vi "uploadProg.vi"(11 "editArray":T1[](array[typedef])) -> (0 "error out":errorcluster)   [LabVIEW 2014]
uses:
  typeDefs/editControl.ctl
  typeDefs/variantFlat.ctl
  typeDefs/pixxelAction.ctl
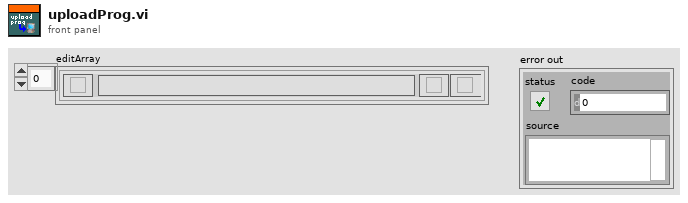
[diagram p1: front panel]
types:
  T1 = typedef "editControl.ctl" = cluster{"edit":bool, "info":string, "variantFlat":T2, "codeCluster":cluster{"code":u8[][]}, "del":bool, "ins":bool}
  T2 = typedef "variantFlat.ctl" = cluster{"type string":i16[], "data string":string}
  T3 = typedef "pixxelAction.ctl" = enum16{"init", "watchdog", "headScene", "setPixel", "tailScene", "headProg", "tailProg", "showSceneFrame", "black", "playFrames", "close", "uploadProg", "startProg", "pauseProg", "stopProg", "jumpTo", "setIP", "setGW", "initFlash", "saveScene", "saveProgram"}
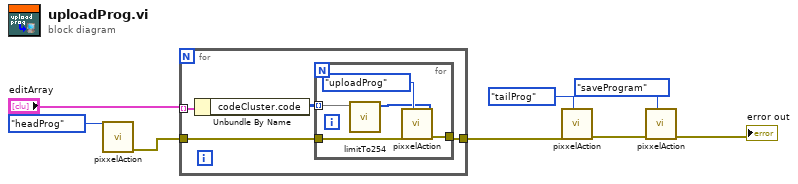
[diagram p0: block diagram]
diagram:
  n1 = call "pixxelAction.vi"("PIXXELaction"=pixxelAction."headProg") -> ("error out"=w5:errorcluster)  [unwired: 10 in]
  n2 = for {
    tunnel: [w12] -> w7
    tunnel: "editArray" -> [w11] mode=indexing
    tunnel: w5 -> [w9]
    n3 = Unbundle By Name(w11) -> ("codeCluster.code"=w10:u8[][])
    n4 = for {
      tunnel: [w17] -> w12
      tunnel: w10 -> [w15] mode=indexing
      tunnel: w9 -> [w13]
      n5 = call "limitTo254.vi"("params"=w15) -> ("limitedTo254"=w14:u8[])  [unwired: 10 in]
      n6 = call "pixxelAction.vi"("inputArray"=w14, "PIXXELaction"=pixxelAction."uploadProg", "error in (no error)"=w13) -> ("error out"=w17:errorcluster)  [unwired: 8 in]
    }
  }
  n7 = call "pixxelAction.vi"("PIXXELaction"=pixxelAction."tailProg", "error in (no error)"=w7) -> ("error out"=w3:errorcluster)  [unwired: 9 in]
  n8 = call "pixxelAction.vi"("PIXXELaction"=pixxelAction."saveProgram", "error in (no error)"=w3) -> ("error out"=→"error out":errorcluster)  [unwired: 9 in]
